vi "buildStartCycle.vi"(8 "error in (no error)":errorcluster, 11 "PlainTextCommandBuilder in":refnum<class "PlainTextCommandBuilder.lvclass">) -> (0 "error out":errorcluster, 2 "message":string, 3 "PlainTextCommandBuilder out":refnum<class "PlainTextCommandBuilder.lvclass">)   [LabVIEW 2023, in "AbstractFactory.lvlib" / "PlainTextCommandBuilder.lvclass"]
uses:
  PlainTextCommandBuilder.lvclass
  PlainTextCommandBuilder.lvclass/PlainTextCommandBuilder.ctl
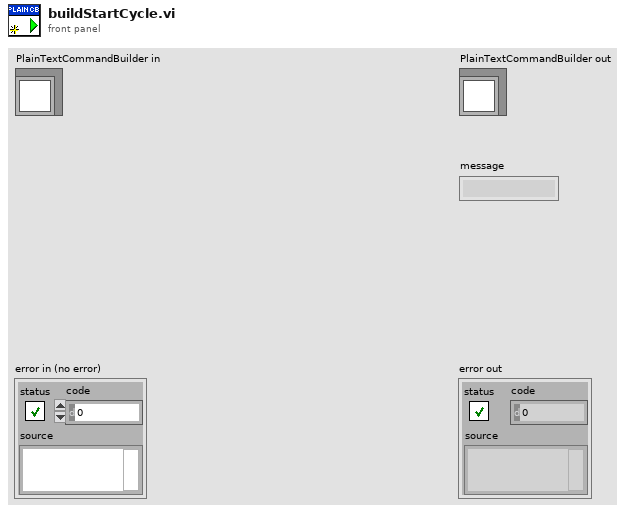
[diagram p1: front panel]
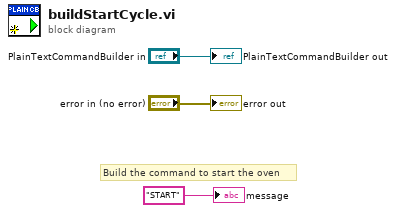
[diagram p0: block diagram]
diagram:
  # "Build the command to start the oven"
  "error out" <- "error in (no error)"
  "PlainTextCommandBuilder out" <- "PlainTextCommandBuilder in"
  "message" <- "START" ("message")
